vi "Gcd.vi"(1 "y":i32, 2 "x":i32) -> (0 "gcd(x,y)":i32)   [LabVIEW 2010, in "NI_Gmath.lvlib"]
doc: "Computes the greatest common divisor of the input values."
uses:
  NI_Gmath.lvlib
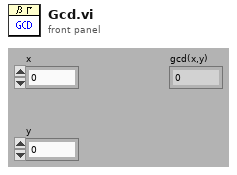
[diagram p1: front panel]
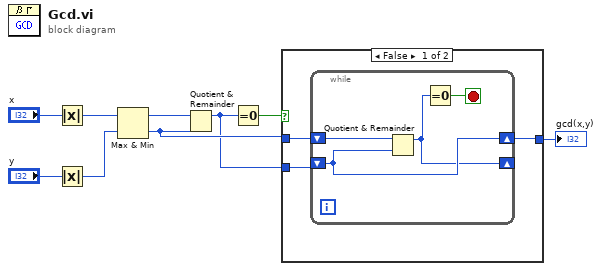
[diagram p0: block diagram]
diagram:
  n1 = Absolute Value(x="x") -> (abs(x)=w3:i32)
  n2 = Absolute Value(x="y") -> (abs(x)=w1:i32)
  n3 = Max & Min(x=w3, y=w1) -> (max(x,y)=w9:i32, min(x,y)=w6:i32)
  n4 = Quotient & Remainder(x=w9, y=w6) -> (x-y*floor(x/y)=w5:i32)  [unwired: 1 out]
  n5 = Equal To 0?(x=w5) -> (x = 0?=w8:bool)
  n6 = case shown="False" w8 {
    tunnel: [w12 w17] -> w7
    tunnel: w6 -> [w11 w17]
    tunnel: w5 -> [w10 _]
    frame False {
      n7 = while {
        shift-right: [w14] -> w12
        shift-left: w11 -> [w15]
        shift-right: [w13] -> _
        shift-left: w10 -> [w14]
        stop <- w16 stop-if-true
        n8 = Quotient & Remainder(x=w15, y=w14) -> (x-y*floor(x/y)=w13:i32)  [unwired: 1 out]
        n9 = Equal To 0?(x=w13) -> (x = 0?=w16:bool)
      }
    }
    frame True {
    }
  }
  "gcd(x,y)" <- w7
